vi "PF2INST.vi"(8 "error in":errorcluster, 9 "Setpoint":dbl, 10 "Run":bool, 11 "Instrument in":refnum<class "Instrument.lvclass">) -> (0 "error out":errorcluster, 3 "Instrument out":refnum<class "Instrument.lvclass">)   [LabVIEW 2019, in "Instrument.lvlib" / "Instrument.lvclass"]
uses:
  Instrument.lvclass
  Instrument.lvclass/Instrument.ctl
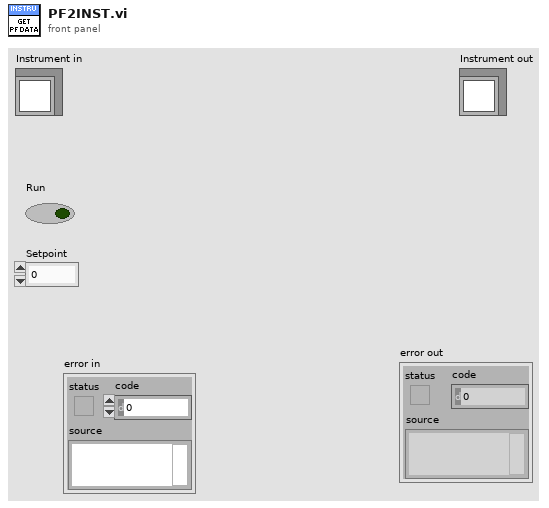
[diagram p1: front panel]
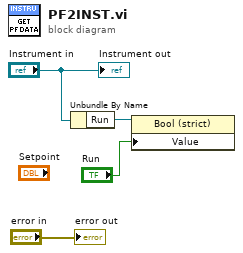
[diagram p0: block diagram]
diagram:
  n1 = Unbundle By Name("Instrument in") -> ("Run"=w2:refnum<vi>)
  n2 = property class="Bool (strict)"(reference=w2, "Value"="Run") -> ()  [unwired: 1 in, 2 out]
  "Instrument out" <- "Instrument in"
  "error out" <- "error in"
